vi "OnEncoderCountChange.vi"(4 "User Parameter":variant, 5 "Event Data":T1, 6 "Control Ref":refnum<k24>, 7 "Event Common Data":T2) -> ()   [LabVIEW 2010]
uses:
  C:/projects/SIMIS/USDigital/QSBLabView2009/USDigital.dll
  projects/SIMIS/USDigital/QSBLabView2009/USDigital.dll
  C:/projects/SIMIS/USDigital/QSBLabView2009/USDQSB.dll
  projects/SIMIS/USDigital/QSBLabView2009/USDQSB.dll
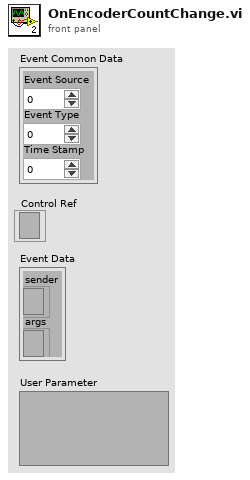
[diagram p1: front panel]
types:
  T1 = cluster{"sender":refnum<k24>, "args":refnum<k24>}
  T2 = cluster{"Event Source":i32, "Event Type":u32, "Time Stamp":u32}
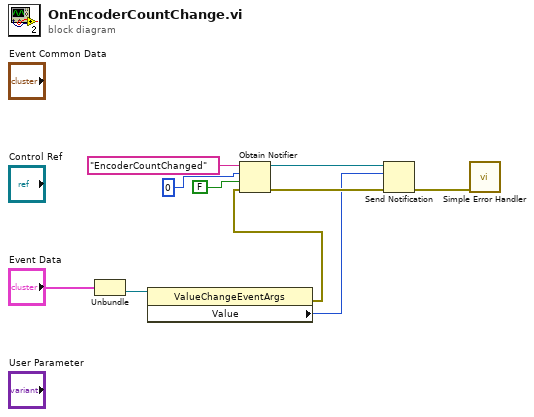
[diagram p0: block diagram]
diagram:
  n1 = Unbundle("Event Data") -> ("args"=w4:refnum<k24>)  [unwired: 1 out]
  n2 = property class="ValueChangeEventArgs"(reference=w4) -> (error out=w2:errorcluster, "Value"=w3:i32)  [unwired: 1 in, 1 out]
  n3 = Obtain Notifier(name (unnamed)="EncoderCountChanged", notification data type=0, create if not found? (T)=FALSE, error in (no error)=w2) -> (notifier out=w7:refnum<notifier>, error out=w6:errorcluster)  [unwired: 1 out]
  n4 = Send Notification(notification=w3, notifier=w7, error in (no error)=w6) -> (error out=w1:errorcluster)  [unwired: 1 out]
  n5 = call <vilib>:"Simple Error Handler.vi"("error in (no error)"=w1) -> ()  [unwired: 4 in, 5 out]
